vi "液压回正判定.vi"(0 "曲线引用":refnum<vi>, 1 "回正判定":T1, 3 "错误输入":errorcluster) -> (7 "曲线引用输出":refnum<vi>, 8 "合格":bool, 10 "错误输出":errorcluster)   [LabVIEW 2018]
uses:
  Global_Variable/Global.vi
  Global_Variable/A180648.vi
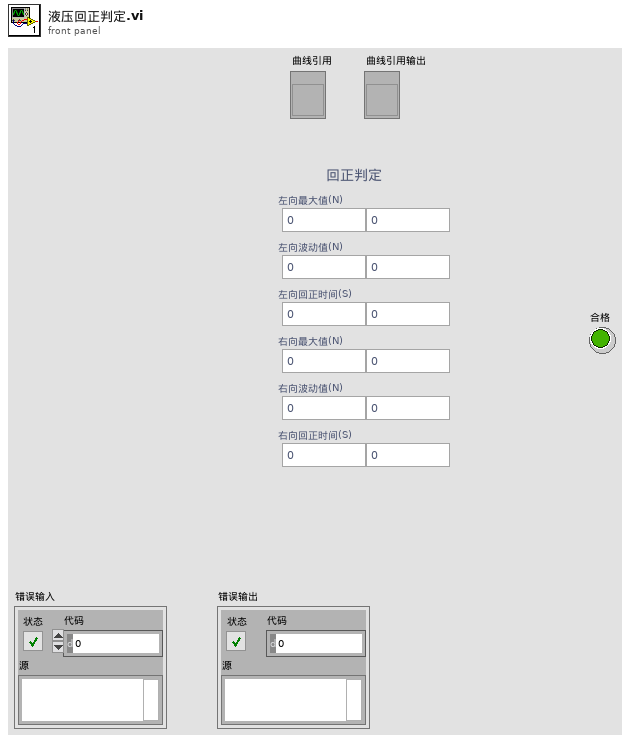
[diagram p1: front panel]
types:
  T1 = cluster{"左向最大值(N)":cluster{"下限":dbl, "上限":dbl}, "左向波动值(N)":cluster{"下限":dbl, "上限":dbl}, "左向回正时间(S)":cluster{"下限":dbl, "上限":dbl}, "右向最大值(N)":cluster{"下限":dbl, "上限":dbl}, "右向波动值(N)":cluster{"下限":dbl, "上限":dbl}, "右向回正时间(S)":cluster{"下限":dbl, "上限":dbl}}
  T2 = enum32{"空载", "功能", "力特性", "传感器特性", "电流特性", "振动NVH", "逆向空载", "完成"}
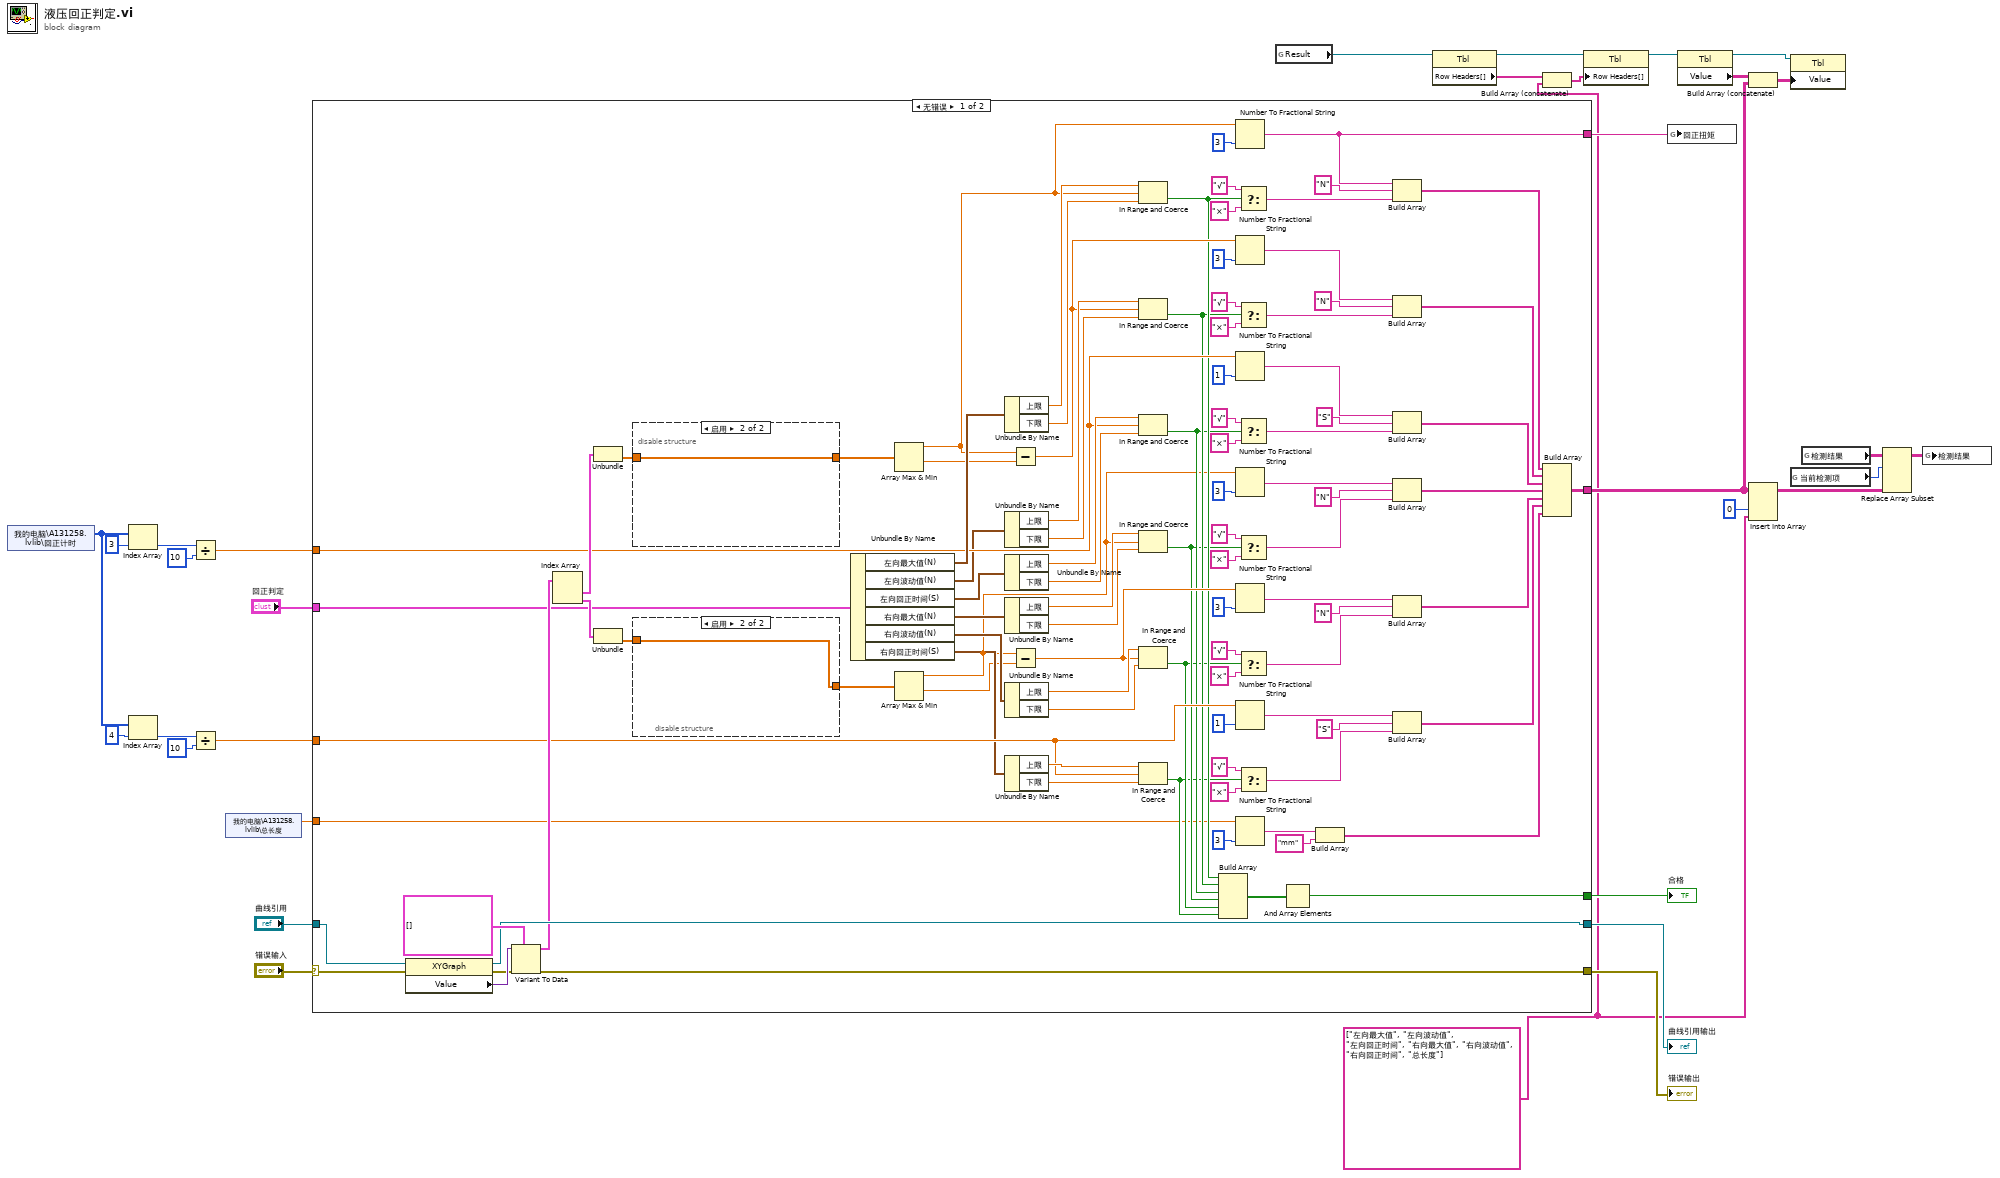
[diagram p0: block diagram]
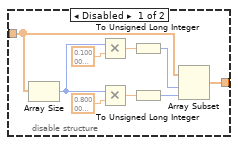
[diagram p2: hidden frame]
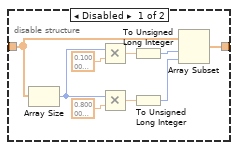
[diagram p3: hidden frame]
diagram:
  w3 = string[] ["左向最大值", "左向波动值", "左向回正时间", "右向最大值", "右向波动值", "右向回正时间", "总长度"] ("元素")
  n1 = shared-variable "我的电脑\\A131258.lvlib\\回正计时"() -> (w21:u32[])  [unwired: 1 in, 1 out]
  n2 = Index Array(array=w21, index=3 ("索引")) -> (element=w19:u32)
  n3 = Index Array(array=w21, index=4 ("索引")) -> (element=w16:u32)
  n4 = Divide(x=w19, y=u32 10) -> (x/y=w20:dbl)
  n5 = Divide(x=w16, y=u32 10) -> (x/y=w15:dbl)
  n6 = shared-variable "我的电脑\\A131258.lvlib\\总长度"() -> (w14:sgl)  [unwired: 1 in, 1 out]
  n7 = case shown="无错误" "错误输入" {
    selector: "错误输入" -> [w127 w151]
    tunnel: [w123 w151] -> w10
    tunnel: "曲线引用" -> [w126 w150]
    tunnel: [w125 w150] -> w13
    tunnel: "回正判定" -> [w119 _]
    tunnel: [w103 _] -> w4
    tunnel: [w98 _] -> w24
    tunnel: w20 -> [w57 _]
    tunnel: w15 -> [w56 _]
    tunnel: w14 -> [w36 _]
    tunnel: [w33 _] -> w8
    frame No Error {
      n8 = property class="XYGraph"(reference=w126, error in=w127) -> (reference out=w125:refnum<vi>, error out=w124:errorcluster, "Value"=w129:variant)
      n9 = Variant To Data(error in=w124, type=cluster{dbl[], dbl[]}[] [], Variant=w129) -> (data=w122:cluster{dbl[], dbl[]}[], error out=w123:errorcluster)
      n10 = Index Array(array=w122) -> (element #1=w121:cluster{dbl[], dbl[]}, element #2=w120:cluster{dbl[], dbl[]})  [unwired: 2 in]
      n11 = Unbundle(w121) -> (w65:dbl[])  [unwired: 1 out]
      n12 = Unbundle(w120) -> (w64:dbl[])  [unwired: 1 out]
      n13 = disable-structure shown="启用" {
        disable-tunnel: [w148 w149] -> w101
        disable-tunnel: w65 -> [w140 w149]
        frame Disabled {
          n14 = Array Size(array=w140) -> (size(s)=w141:i32)
          n15 = Multiply(x=w141, y=sgl 0.1) -> (x*y=w145:sgl)
          n16 = Multiply(x=w141, y=sgl 0.8) -> (x*y=w146:sgl)
          n17 = To Unsigned Long Integer(number=w145) -> (unsigned 32bit integer=w147:u32)
          n18 = To Unsigned Long Integer(number=w146) -> (unsigned 32bit integer=w142:u32)
          n19 = Array Subset(array=w140, index=w147, length=w142) -> (w148:dbl[])
        }
        frame Enabled {
        }
      }
      n20 = disable-structure shown="启用" {
        disable-tunnel: [w138 w139] -> w102
        disable-tunnel: w64 -> [w130 w139]
        frame Disabled {
          n21 = Array Size(array=w130) -> (size(s)=w137:i32)
          n22 = Multiply(x=w137, y=sgl 0.1) -> (x*y=w133:sgl)
          n23 = Multiply(x=w137, y=sgl 0.8) -> (x*y=w132:sgl)
          n24 = To Unsigned Long Integer(number=w133) -> (unsigned 32bit integer=w131:u32)
          n25 = To Unsigned Long Integer(number=w132) -> (unsigned 32bit integer=w136:u32)
          n26 = Array Subset(array=w130, index=w131, length=w136) -> (w138:dbl[])
        }
        frame Enabled {
        }
      }
      n27 = Unbundle By Name(w119) -> ("左向最大值(N)"=w118:cluster{"下限":dbl, "上限":dbl}, "左向波动值(N)"=w55:cluster{"下限":dbl, "上限":dbl}, "左向回正时间(S)"=w54:cluster{"下限":dbl, "上限":dbl}, "右向最大值(N)"=w63:cluster{"下限":dbl, "上限":dbl}, "右向波动值(N)"=w53:cluster{"下限":dbl, "上限":dbl}, "右向回正时间(S)"=w52:cluster{"下限":dbl, "上限":dbl})
      n28 = Array Max & Min(array=w101) -> (max value=w62:dbl, min value=w61:dbl)  [unwired: 2 out]
      n29 = Array Max & Min(array=w102) -> (max value=w34:dbl, min value=w51:dbl)  [unwired: 2 out]
      n30 = Unbundle By Name(w118) -> ("上限"=w105:dbl, "下限"=w104:dbl)
      n31 = Unbundle By Name(w55) -> ("上限"=w95:dbl, "下限"=w96:dbl)
      n32 = Unbundle By Name(w54) -> ("上限"=w84:dbl, "下限"=w83:dbl)
      n33 = Unbundle By Name(w63) -> ("上限"=w100:dbl, "下限"=w99:dbl)
      n34 = Unbundle By Name(w53) -> ("上限"=w80:dbl, "下限"=w81:dbl)
      n35 = Unbundle By Name(w52) -> ("上限"=w67:dbl, "下限"=w66:dbl)
      n36 = Subtract(x=w62, y=w61) -> (x-y=w60:dbl)
      n37 = Subtract(x=w34, y=w51) -> (x-y=w50:dbl)
      n38 = In Range and Coerce(upper limit=w105, x=w62, lower limit=w104) -> (In Range?=w45:bool)  [unwired: 1 out]
      n39 = In Range and Coerce(upper limit=w95, x=w60, lower limit=w96) -> (In Range?=w44:bool)  [unwired: 1 out]
      n40 = In Range and Coerce(upper limit=w84, x=w57, lower limit=w83) -> (In Range?=w43:bool)  [unwired: 1 out]
      n41 = In Range and Coerce(upper limit=w100, x=w34, lower limit=w99) -> (In Range?=w42:bool)  [unwired: 1 out]
      n42 = In Range and Coerce(upper limit=w80, x=w50, lower limit=w81) -> (In Range?=w41:bool)  [unwired: 1 out]
      n43 = In Range and Coerce(upper limit=w67, x=w56, lower limit=w66) -> (In Range?=w40:bool)  [unwired: 1 out]
      n44 = Build Array(w45, w44, w43, w42, w41, w40) -> (w106:bool[])
      n45 = Number To Fractional String(number=w62, precision (6)=i16 3 ("精度(6)")) -> (F-format string=w98:string)  [unwired: 2 in]
      n46 = Number To Fractional String(number=w60, precision (6)=i16 3 ("精度(6)")) -> (F-format string=w97:string)  [unwired: 2 in]
      n47 = Number To Fractional String(number=w57, precision (6)=i16 1 ("精度(6)")) -> (F-format string=w82:string)  [unwired: 2 in]
      n48 = Number To Fractional String(number=w34, precision (6)=i16 3 ("精度(6)")) -> (F-format string=w108:string)  [unwired: 2 in]
      n49 = Number To Fractional String(number=w50, precision (6)=i16 3 ("精度(6)")) -> (F-format string=w78:string)  [unwired: 2 in]
      n50 = Number To Fractional String(number=w56, precision (6)=i16 1 ("精度(6)")) -> (F-format string=w69:string)  [unwired: 2 in]
      n51 = Number To Fractional String(number=w36, precision (6)=i16 3 ("精度(6)")) -> (F-format string=w38:string)  [unwired: 2 in]
      n52 = Select(t="√", s=w45, f="×") -> (s? t:f=w113:string)
      n53 = Select(t="√", s=w44, f="×") -> (s? t:f=w94:string)
      n54 = Select(t="√", s=w43, f="×") -> (s? t:f=w85:string)
      n55 = Select(t="√", s=w42, f="×") -> (s? t:f=w112:string)
      n56 = Select(t="√", s=w41, f="×") -> (s? t:f=w74:string)
      n57 = Select(t="√", s=w40, f="×") -> (s? t:f=w73:string)
      n58 = And Array Elements(Boolean array=w106) -> (logical AND=w33:bool)
      n59 = Build Array(w38, "mm" ("元素")) -> (w35:string[])
      n60 = Build Array(w98, "N" ("元素"), w113) -> (w59:string[])
      n61 = Build Array(w97, "N" ("元素"), w94) -> (w58:string[])
      n62 = Build Array(w82, "S" ("元素"), w85) -> (w49:string[])
      n63 = Build Array(w108, "N" ("元素"), w112) -> (w48:string[])
      n64 = Build Array(w78, "N" ("元素"), w74) -> (w47:string[])
      n65 = Build Array(w69, "S" ("元素"), w73) -> (w46:string[])
      n66 = Build Array(w59, w58, w49, w48, w47, w46, w35) -> (w103:string[][])
    }
    frame Error {
    }
  }
  "错误输出" <- w10
  "曲线引用输出" <- w13
  "合格" <- w8
  n67 = global read "Global.vi" "Result"() -> (w32:refnum<vi>)
  n68 = property class="Tbl"(reference=w32) -> (reference out=w29:refnum<vi>, "Row Headers[]"=w31:string[])  [unwired: 1 in, 1 out]
  n69 = Build Array (concatenate)(w31, w3) -> (w30:string[])
  n70 = property class="Tbl"(reference=w29, "Row Headers[]"=w30) -> (reference out=w28:refnum<vi>)  [unwired: 1 in, 1 out]
  n71 = global write "检测结果.vi" "回正扭矩"(w24) -> ()
  n72 = property class="Tbl"(reference=w28) -> (reference out=w27:refnum<vi>, "Value"=w26:string[][])  [unwired: 1 in, 1 out]
  n73 = Build Array (concatenate)(w26, w4) -> (w25:string[][])
  n74 = Insert Into Array(array=w4, index (col)=0 ("禁用的索引 (列)"), new element=w3) -> (w1:string[][])  [unwired: 1 in]
  n75 = property class="Tbl"(reference=w27, "Value"=w25) -> ()  [unwired: 1 in, 2 out]
  n76 = global read "A180648.vi" "当前检测项"() -> (w6:T2)
  n77 = global read "A180648.vi" "检测结果"() -> (w7:string[][][])
  n78 = Replace Array Subset(array=w7, new element=w1, index (dim 0)=w6) -> (w5:string[][][])  [unwired: 2 in]
  n79 = global write "A180648.vi" "检测结果"(w5) -> ()
